vi "Check Leakage.vi"(8 "error in":errorcluster, 11 "BoardHandle in":T1) -> (0 "error out":errorcluster, 1 "Ch1 Leak":dbl, 2 "Ch0 Leak":dbl, 3 "BoardHandle out":T1)   [LabVIEW 2020]
uses:
  <instrlib>/CAEN PSM/CAEN PSM.lvlib
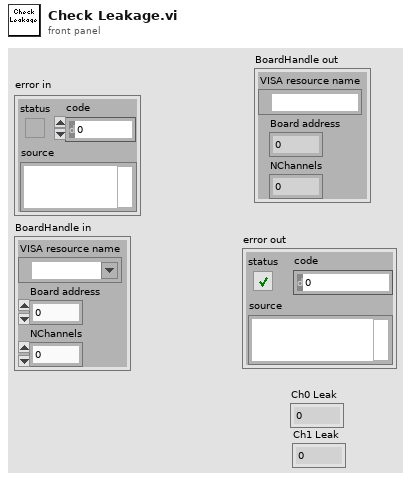
[diagram p1: front panel]
types:
  T1 = cluster{"VISA resource name":refnum<visa-resource-name>, "Board address":u8, "NChannels":u8}
  T2 = typedef "CAEN PSM.lvlib/BoardHandle.ctl" = cluster{"VISA resource name":refnum<visa-resource-name>, "Board address":i8, "NChannels":u8}
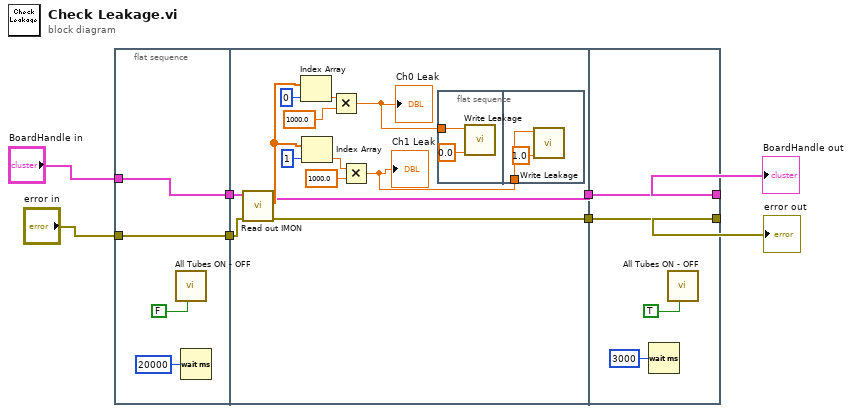
[diagram p0: block diagram]
diagram:
  n1 = flat-sequence {
    tunnel: "BoardHandle in" -> [w11]
    tunnel: "error in" -> [w10]
    tunnel: [w11] -> w2
    tunnel: [w10] -> w1
    tunnel: [w15] -> w4
    tunnel: [w16] -> w3
    tunnel: w2 -> [w18]
    tunnel: w1 -> [w17]
    tunnel: [w32] -> w5
    tunnel: [w33] -> w6
    tunnel: w4 -> [w33]
    tunnel: w3 -> [w32]
    frame #0 {
      n2 = call "All Tubes ON - OFF.vi"("Tubes ON/OFF"=FALSE) -> ()  [unwired: 11 in]
      n3 = Wait (ms)(milliseconds to wait=u32 20000) -> ()  [unwired: 1 out]
    }
    frame #1 {
      n4 = call <instrlib>:"Read out IMON.vi"("error in (no error)"=w17, "BoardHandle"=w18) -> ("error out"=w16:errorcluster, "IMon values (uA)"=w23:dbl[], "BoardHandle out"=w15:T2)  [unwired: 6 in, 1 out]
      n5 = Index Array(array=w23, index=0) -> (element=w22:dbl)
      n6 = Index Array(array=w23, index=1) -> (element=w20:dbl)
      n7 = Multiply(x=w22, y=1000.0) -> (x*y=w14:dbl)
      "Ch0 Leak" <- w14
      n8 = Multiply(x=w20, y=1000.0) -> (x*y=w13:dbl)
      "Ch1 Leak" <- w13
      n9 = flat-sequence {
        tunnel: w14 -> [w27]
        tunnel: w13 -> [w28]
        frame #0 {
          n10 = call "Write Leakage.vi"("Channel #"=0.0, "Leakage"=w27) -> ()  [unwired: 10 in]
        }
        frame #1 {
          n11 = call "Write Leakage.vi"("Channel #"=1.0, "Leakage"=w28) -> ()  [unwired: 10 in]
        }
      }
    }
    frame #2 {
      n12 = Wait (ms)(milliseconds to wait=u32 3000) -> ()  [unwired: 1 out]
      n13 = call "All Tubes ON - OFF.vi"("Tubes ON/OFF"=TRUE) -> ()  [unwired: 11 in]
    }
  }
  "BoardHandle out" <- w6
  "error out" <- w5
